vi "__YIG_OSC_6501.vi"(0 "fc(GHz)":dbl=23.0, 2 "bit":i32=8, 3 "Dev(1,2..)":i32=2) -> ()   [LabVIEW 2017]
panel:
  out "設定値":i32 format="%x"
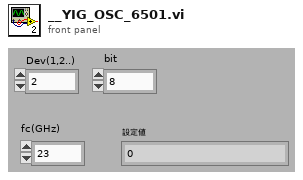
[diagram p1: front panel]
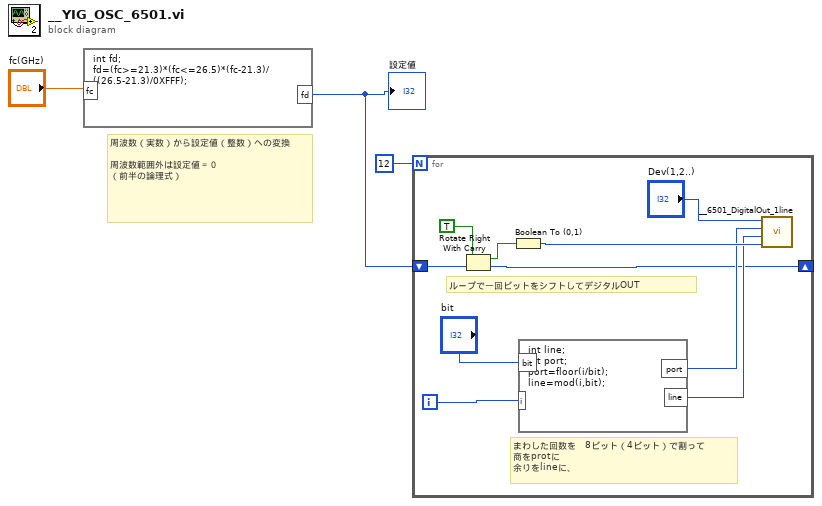
[diagram p0: block diagram]
diagram:
  # "周波数（実数）から設定値（整数）への変換 \n\n周波数範囲外は設定値＝０\n（前半の論理式）"
  n1 = formula code="int fd;\nfd=(fc>=21.3)*(fc<=26.5)*(fc-21.3)/((26.5-21.3)/0XFFF);"("fc"="fc(GHz)") -> ("fd"=w2:i32)
  "設定値" <- w2
  n2 = for {
    N: 12 -> [_]
    shift-right: [w4] -> _
    shift-left: w2 -> [w13]
    i -> [w8]
    # "ループで一回ビットをシフトしてデジタルOUT"
    # "まわした回数を　8ビット（4ビット）で割って\n商をprotに\n余りをlineに、"
    n3 = Rotate Right With Carry(2:w13, 3:TRUE) -> (0:w4:i32, 1:w12:bool)
    n4 = Boolean To (0,1)(Boolean=w12) -> (0, 1=w11:i16)
    n5 = formula code="int line;\nint port;\nport=floor(i/bit);\nline=mod(i,bit);"("bit"="bit", "i"=w8) -> ("line"=w6:i32, "port"=w5:i32)
    n6 = call "__6501_DigitalOut_1line.vi"("OFF,ON(0,1)"=w11, "line(0...7)"=w6, "Port(0,1,2)"=w5, "Dev(1,2..)"="Dev(1,2..)") -> ()
  }
